vi "Main.vi"() -> ()   [LabVIEW 2015]
uses:
  <vilib>/sound2/lvsound2.llb/Sampling Mode.ctl
  <vilib>/sound2/lvsound2.llb/Sound Data Format.ctl
  <vilib>/sound2/lvsound2.llb/Sound Output Set Volume (Single).vi
  <vilib>/sound2/lvsound2.llb/Sound Output Write (DBL Single).vi
  <vilib>/measure/NI_MABase.lvlib
panel:
  in  "System Start Button":bool
  in  "Vertical Cancel Button 2":bool
  in  "Pict Ring":u16(ring)
  in  "Volume":dbl(slide) scale=0.0..100.0
  in  "Dial":dbl(knob)=1.0 min=1.0 max=20000.0 scale=1.0..20000.0
  # "Frequency Generator"
  # "Frequency"
  # "Hz"
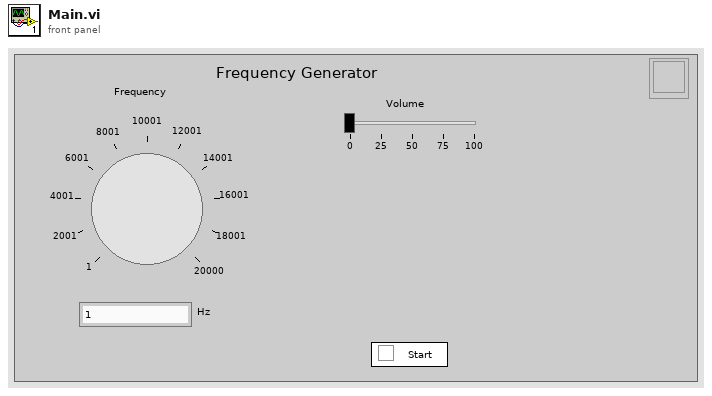
[diagram p1: front panel]
types:
  T1 = enum8{"Enabled", "Disabled", "Disabled and Grayed Out"}
  T2 = typedef "Sound Data Format.ctl" = cluster{"sample rate (S/s)":dbl, "number of channels":i32, "bits per sample":i32}
  T3 = enum16{"Sine Wave", "Triangle Wave", "Square Wave", "Sawtooth Wave"}
  T4 = typedef "Sampling Mode.ctl" = i32
  T5 = typedef "Sound Output Task ID.ctl" = u32
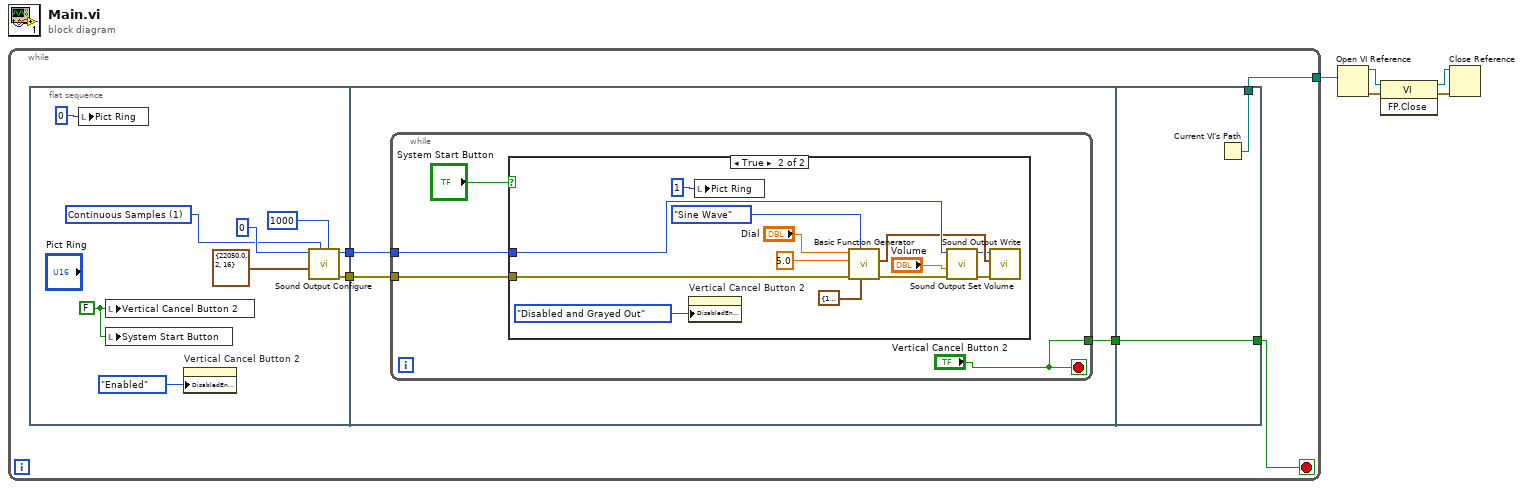
[diagram p0: block diagram]
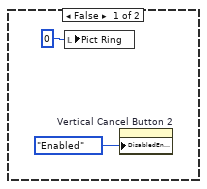
[diagram p2: hidden frame]
diagram:
  n1 = while {
    tunnel: [w8] -> w5
    stop <- w6 stop-if-true
    n2 = flat-sequence {
      tunnel: [w14] -> w10
      tunnel: [w13] -> w9
      tunnel: w10 -> [w22]
      tunnel: w9 -> [w21]
      tunnel: [w20] -> w7
      tunnel: [w43] -> w8
      tunnel: w7 -> [w42]
      tunnel: [w42] -> w6
      frame #0 {
        w12 = FALSE ("Vertical Cancel Button")
        w15 = T4 1 items=["Finite Samples", "Continuous Samples"] ("sample mode")
        n3 = local write "Pict Ring"(u16 0 ("Pict Ring")) -> ()
        n4 = local write "Vertical Cancel Button 2"(w12) -> ()
        n5 = local write "System Start Button"(w12) -> ()
        n6 = property on="Vertical Cancel Button 2" class="Bool (strict)"("DisabledEnum"=T1."Enabled" ("Disabled")) -> ()  [unwired: 2 in, 2 out]
        n7 = call <vilib>:"Sound Output Configure.vi"("number of samples/ch"=1000, "sample mode"=w15, "sound format"=T2 {"sample rate (S/s)"=22050.0, "number of channels"=2, "bits per sample"=16}, "device ID"=u32 0) -> ("error out"=w13:errorcluster, "task ID"=w14:T5)  [unwired: 6 in]
      }
      frame #1 {
        n8 = while {
          tunnel: w22 -> [w25]
          tunnel: w21 -> [w24]
          tunnel: ["Vertical Cancel Button 2"] -> w20
          stop <- "Vertical Cancel Button 2" stop-if-true
          n9 = case shown="True" "System Start Button" {
            tunnel: w25 -> [_ w41]
            tunnel: w24 -> [_ w40]
            frame False {
              n10 = local write "Pict Ring"(u16 0 ("Pict Ring")) -> ()
              n11 = property on="Vertical Cancel Button 2" class="Bool (strict)"("DisabledEnum"=T1."Enabled" ("Disabled")) -> ()  [unwired: 2 in, 2 out]
            }
            frame True {
              n12 = property on="Vertical Cancel Button 2" class="Bool (strict)"("DisabledEnum"=T1."Disabled and Grayed Out" ("Disabled")) -> ()  [unwired: 2 in, 2 out]
              n13 = local write "Pict Ring"(u16 1 ("Pict Ring")) -> ()
              n14 = call <vilib>:"Basic Function Generator.vi"("sampling info"=cluster{"Fs":dbl, "#s":dbl} {"Fs"=100000.0, "#s"=100000.0}, "signal type"=T3."Sine Wave", "error in (no error)"=w40, "amplitude"=5.0, "frequency"="Dial") -> ("error out"=w30:errorcluster, "signal out"=w36:waveform(dbl))  [unwired: 4 in, 1 out]
              n15 = call-poly <vilib>:"Sound Output Set Volume.vi"("error in (no error)"=w30, "volume"="Volume", "task ID"=w41) -> ("error out"=w32:errorcluster, "task ID out"=w33:T5)  [unwired: 7 in]
              n16 = call-poly <vilib>:"Sound Output Write.vi"("error in (no error)"=w32, "data"=w36, "task ID"=w33) -> ()  [unwired: 7 in, 2 out]
            }
          }
        }
      }
      frame #2 {
        n17 = Current VI's Path() -> (path=w43:path)
      }
    }
  }
  n18 = Open VI Reference(vi path=w5) -> (vi reference=w4:refnum<vi>, error out=w3:errorcluster)  [unwired: 5 in]
  n19 = invoke class="VI" method="FP.Close"(reference=w4, error in=w3) -> (reference out=w2:refnum<vi>, error out=w1:errorcluster)  [unwired: 1 in, 1 out]
  n20 = Close Reference(reference=w2, error in (no error)=w1) -> ()  [unwired: 1 out]
